vi "zmq_ctx_create.vi"(3 "error in":errorcluster) -> (0 "error out":errorcluster, 2 "context out":refnum<class "zmq_context.lvclass">)   [LabVIEW 2019, in "zeromq.lvlib" / "zmq_context.lvclass"]
doc: "Instantiate ZeroMQ and return a <b>context</b> to create sockets with. Ideally, this should only be called once per application and the context shared.\n\nPreviously called <b>zmq_init</b>.\n\nDetailed API documentation: http://api.zeromq.org/3-2:zmq-ctx-new"
uses:
  zmq_context.lvclass
  zmq_context.lvclass/zmq_context.ctl
  <vilib>/Utility/error.llb/Error Cluster From Error Code.vi
  zeromq.lvlib
panel:
  # "ØMQ"
  # "labview"
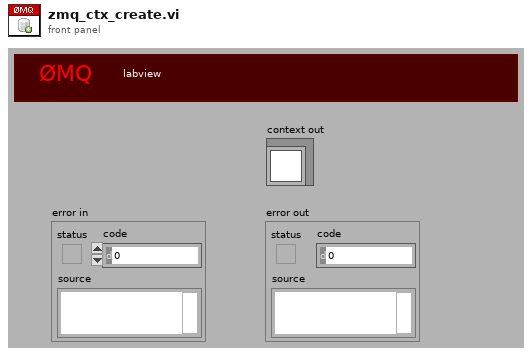
[diagram p1: front panel]
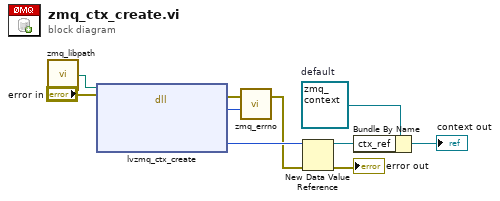
[diagram p0: block diagram]
diagram:
  w9 = refnum<class "zmq_context.lvclass"> refnum  # default
  n1 = call "zmq_libpath.vi"() -> ("path"=w1:path)
  n2 = dll-call lib="?" fn="lvzmq_ctx_create" ("zmq_labview.dll:lvzmq_init")(path in=w1, error in="error in") -> (error out=w7:errorcluster, "return value"=w6:i32, "ctx_obj"=w5:u64)  [unwired: 4 in, 1 out]
  n3 = call "zmq_errno.vi"("retval"=w6, "error in"=w7) -> ("error out"=w4:errorcluster)  [unwired: 1 out]
  n4 = New Data Value Reference(data value=w5, error in=w4) -> (data value reference=w3:refnum<data-value>, error out=→"error out":errorcluster)
  n5 = Bundle By Name(cluster=w9, "ctx_ref"=w3) -> (→"context out":refnum<class "zmq_context.lvclass">)
